vi "LimitAmp.vi"(8 "data in":dbl, 11 "limit":dbl) -> (0 "data out":dbl)   [LabVIEW 2020]
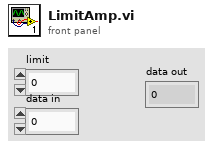
[diagram p1: front panel]
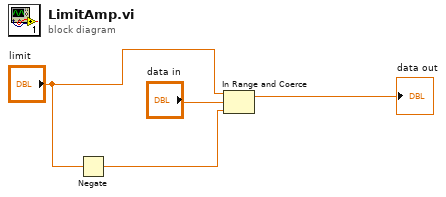
[diagram p0: block diagram]
diagram:
  n1 = Negate(x="limit") -> (-x=w4:dbl)
  n2 = In Range and Coerce(upper limit="limit", x="data in", lower limit=w4) -> (coerced(x)=→"data out":dbl)  [unwired: 1 out]
